vi "Cluster-Array.vi"(5 "error in":errorcluster, 8 "data":cluster{"table":string, dbl, dbl}[](array[cluster])) -> (0 "error out":errorcluster, 1 "V2":dbl[](array[numeric]), 2 "V1":dbl[](array[numeric]), 3 "tiempo":timestamp[](array[timestamp]) format="%<%I:%M:%S %p\n%d/%m/%y>T")   [LabVIEW 2020]
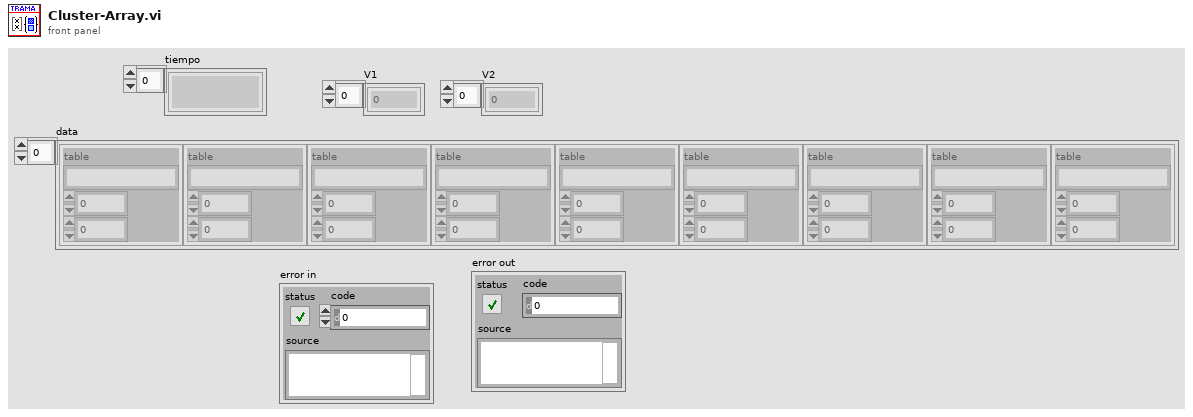
[diagram p1: front panel]
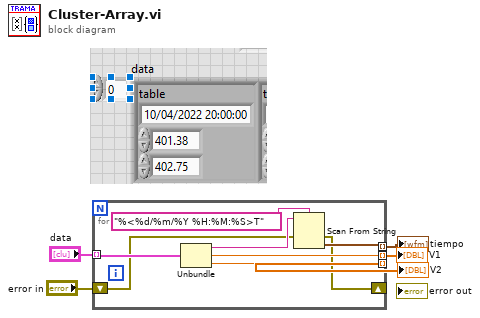
[diagram p0: block diagram]
diagram:
  n1 = for {
    tunnel: "data" -> [w13] mode=indexing
    tunnel: [w12] -> w4 mode=indexing
    tunnel: [w11] -> w3 mode=indexing
    tunnel: [w9] -> w2 mode=indexing
    shift-right: [w6] -> _
    shift-left: "error in" -> [w7]
    n2 = Unbundle(w13) -> ("table"=w10:string, w12:dbl, w11:dbl)
    n3 = Scan From String(format string="%<%d/%m/%Y %H:%M:%S>T", input string=w10, error in=w7) -> (error out=w6:errorcluster, output 1=w9:timestamp)  [unwired: 2 in, 2 out]
  }
  "V1" <- w4
  "V2" <- w3
  "tiempo" <- w2
